vi "Analog Input - 1 Channel - 1 Sample.vi"() -> ()   [LabVIEW 2019]
uses:
  <vilib>/myRIO/Common/Instrument Driver Framework/ELVIS III v1.0/AI/vis/ELVIS III v1.0 Close AI.vi
  <vilib>/myRIO/Common/Instrument Driver Framework/myRIO v1.0/UART/vis/myRIO v1.0 Close UART.vi
  <vilib>/myRIO/Common/Instrument Driver Framework/ELVIS III v1.0/AI/vis/ELVIS III v1.0 Unreserve AI.vi
  <vilib>/myRIO/Common/Instrument Driver Framework/ELVIS III v1.0/AI/vis/ELVIS III v1.0 Build MUX Configuration AI.vi
  <vilib>/Utility/error.llb/Error Cluster From Error Code.vi
  <vilib>/myRIO/Common/Instrument Driver Framework/ELVIS III v1.0/AI/vis/ELVIS III v1.0 Read AI.vi
  <vilib>/myRIO/Common/Instrument Driver Framework/ELVIS III v1.0/Resource Manager/vis/ELVIS III v1.0 Unreserve Channel List.vi
  <vilib>/myRIO/Common/Instrument Driver Framework/myRIO v1.0/myRIO v1.0 Close.vi
  <vilib>/myRIO/Common/Instrument Driver Framework/Utilities/vis/FPGA Ref Manager.vi
  <vilib>/myRIO/Common/Instrument Driver Framework/ELVIS III v1.0/ELVIS III v1.0 Reset FPGA.vi
  <vilib>/myRIO/Common/Instrument Driver Framework/myRIO v1.0/IRQ/vis/myRIO v1.0 IRQ Info FGV.vi
  <vilib>/myRIO/Common/Instrument Driver Framework/myRIO v1.0/IRQ/vis/myRIO v1.0 Timer IRQ Info FGV.vi
  <vilib>/myRIO/Common/Instrument Driver Framework/myRIO v1.0/IRQ/vis/myRIO v1.0 ISR Agent.vi
  <vilib>/myRIO/Instrument Drivers/Utilities/vis/Reset Index.vi
  <vilib>/myRIO/Common/Instrument Driver Framework/myRIO v1.0/Resource Manager/vis/myRIO v1.0 Block Write Resource Manager.vi
  <vilib>/myRIO/Instrument Drivers/Utilities/Utilities.lvlib
  <vilib>/myRIO/Instrument Drivers/Onboard IO/AI/AI.lvlib
panel:
  out "Analog Data":dbl(graph)
  in  "Stop":bool
  # "ELVIS III Control IO"
  # "模拟输入"
  # "Overview: Acquires single point voltage values each loop iteration from Bank A, Channel 0 (A/AI0).\nInstructions:\n1. Connect A/AI0 to a valid signal.\n2. Run the VI."
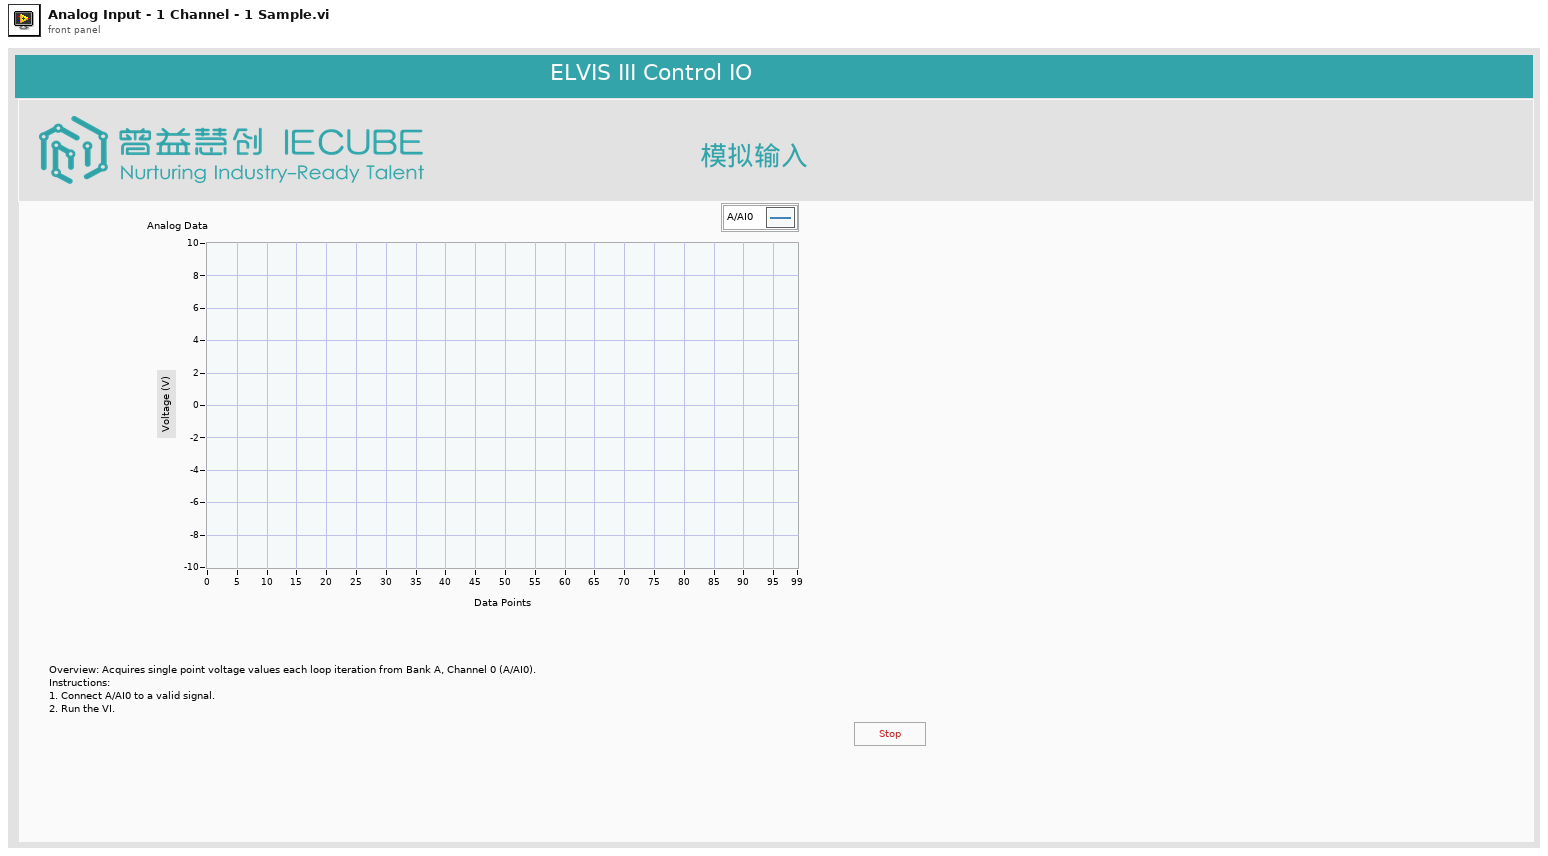
[diagram p1: front panel]
types:
  T1 = typedef "AI.lvlib/AI Reference.ctl" = cluster{"myRIO Reference":T2, "AI Channels List":T6, "AI Scaling Constants List":T8}
  T2 = typedef "myRIO Generic Hardware Reference.ctl" = cluster{"myRIO Model":T3, "myRIO Hardware Reference":T4}
  T3 = typedef "Hardware Version Enum.ctl" = enum16{"Unknown", "myRIO-1900", "myRIO-1950", "roboRIO", "NI ELVIS RIO CM", "ELVIS III"}
  T4 = typedef "myRIO v1.0 Reference.ctl" = cluster{"Generic FPGA Reference":T5, "Allow multiple opens":bool}
  T5 = typedef "Generic FPGA Reference.ctl" = refnum<k20>
  T6 = typedef "AI Channels List.ctl" = T7[]
  T7 = typedef "AI Channels Enum.ctl" = enum16{"Not Connected", "AudioIn/Left", "AudioIn/Right", "C/AI0", "C/AI1", "A/AI0", "A/AI1", "A/AI2", "A/AI3", "A/AI4", "A/AI5", "A/AI6", "A/AI7", "B/AI0", "B/AI1", "B/AI2", "B/AI3", "B/AI4", "B/AI5", "B/AI6", "B/AI7", "AI/AI0", "AI/AI1", "AI/AI2", "AI/AI3", "A/AI0 (DIFF)", "A/AI1 (DIFF)", "A/AI2 (DIFF)", "A/AI3 (DIFF)", "B/AI0 (DIFF)", "B/AI1 (DIFF)", "B/AI2 (DIFF)", "B/AI3 (DIFF)"}
  T8 = typedef "Analog Scaling Constants List.ctl" = T9[]
  T9 = typedef "Analog Scaling Constants.ctl" = cluster{"LSB Weight (Volts)":dbl, "Offset (Volts)":dbl, "Signed?":bool}
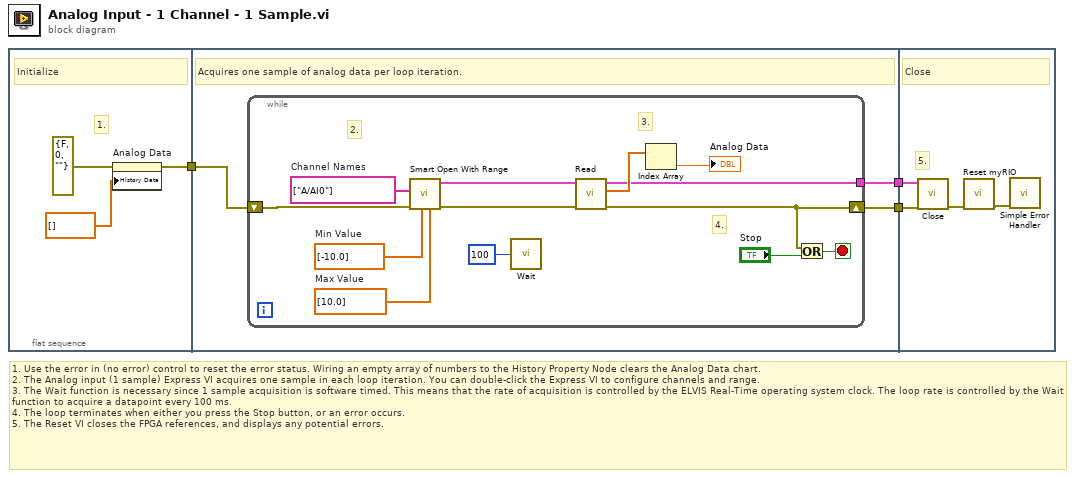
[diagram p0: block diagram]
diagram:
  # "1. Use the error in (no error) control to reset the error status. Wiring an empty array of numbers to the History Property Node clears the Analog Data chart.\n2. The Analog input (1 sample) Express VI acquires one sample in each loop iteration. You can double-click the Express VI to configure channels and range.\n3. The Wait function is necessary since 1 sample acquisition is software timed. This means that the rate of acquisition is controlled by the ELVIS Real-Time operating system clock. The loop rate is controlled by the Wait function to acquire a datapoint every 100 ms.\n4. The loop terminates when either you press the Stop button, or an error occurs.\n5. The Reset VI closes the FPGA references, and displays any potential errors."
  n1 = flat-sequence {
    tunnel: [w6] -> w3
    tunnel: w3 -> [w9]
    tunnel: [w8] -> w2
    tunnel: [w7] -> w1
    tunnel: w2 -> [w24]
    tunnel: w1 -> [w25]
    frame #0 {
      # "1."
      # "Initialize"
      n2 = property on="Analog Data" class="WFChart (严格)"(error in=errorcluster {"status"=FALSE, "code"=0, "source"=""} ("error in (no error)"), "History Data"=dbl[] []) -> (error out=w6:errorcluster)  [unwired: 1 in, 1 out]
    }
    frame #1 {
      # "Acquires one sample of analog data per loop iteration."
      n3 = while {
        shift-right: [w13] -> w8
        shift-left: w9 -> [w15]
        tunnel: [w10] -> w7
        stop <- w22 stop-if-true
        w11 = dbl[] [10.0]  # Max Value
        w12 = dbl[] [-10.0]  # Min Value
        w16 = tag[] ["A/AI0"]  # Channel Names
        # "4."
        # "3."
        # "2."
        n4 = call <vilib>:"Smart Open With Range.vi"("Max Value"=w11, "Min Value"=w12, "error in (no error)"=w15, "Channel Names"=w16) -> ("error out"=w19:errorcluster, "AI Ref Out"=w18:T1)  [unwired: 6 in]
        n5 = call "Wait"("Count(mSec)"=u32 100) -> ()  [unwired: 1 out]
        n6 = call <vilib>:"Read.vi"("error in (no error)"=w19, "AI Ref In"=w18) -> ("error out"=w13:errorcluster, "Values"=w17:dbl[], "AI Ref Out"=w10:T1)  [unwired: 7 in]
        n7 = Index Array(array=w17) -> (element=→"Analog Data":dbl)  [unwired: 1 in]
        n8 = Or(x=w13, y="Stop") -> (x .or. y?=w22:bool)
      }
    }
    frame #2 {
      # "5."
      # "Close"
      n9 = call <vilib>:"Close.vi"("error in (no error)"=w24, "AI Ref In"=w25) -> ("error out"=w23:errorcluster)  [unwired: 9 in]
      n10 = call <vilib>:"Reset myRIO.vi"("error in (no error)"=w23) -> ("error out"=w26:errorcluster)  [unwired: 10 in]
      n11 = call <vilib>:"Simple Error Handler.vi"("error in (no error)"=w26) -> ()  [unwired: 4 in, 5 out]
    }
  }
